vi "nominal workbook create commit.vi"(7 "out_workbook":i32, 8 "error in (no error)":errorcluster, 9 "staging":i32, 10 "template_":i32, 11 "client":i32) -> (0 "error out":errorcluster, 3 "function return":i32, 5 "out_workbook out":i32)   [LabVIEW 2020, in "client.lvlib"]
doc: "int32_t nominal_workbook_create_commit(int32_t client,\n int32_t template_,\n int32_t staging,\n int32_t *out_workbook);"
uses:
  client.lvlib
  bin/nominalClient_64.dll
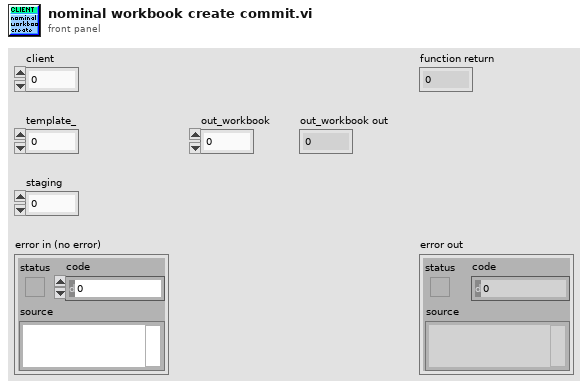
[diagram p1: front panel]
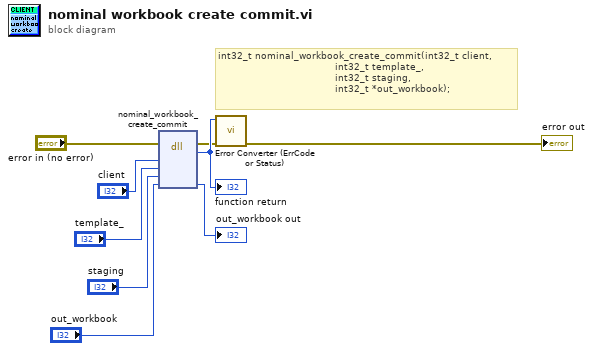
[diagram p0: block diagram]
diagram:
  # "int32_t nominal_workbook_create_commit(int32_t client,\n                                       int32_t template_,\n                                       int32_t staging,\n                                       int32_t *out_workbook);"
  n1 = dll-call lib="C:/code/labview-client-rs/lv_src/bin/nominalClient_*.*" fn="nominal_workbook_create_commit"(error in="error in (no error)", "client"="client", "template_"="template_", "staging"="staging", "out_workbook"="out_workbook") -> (error out=w2:errorcluster, w9:i32, "out_workbook"=→"out_workbook out":i32)  [unwired: 5 in, 1 out]
  "function return" <- w9
  n2 = call "Error Converter (ErrCode or Status).vi"("error in (no error)"=w2, "error code"=w9) -> ("error out"=→"error out":errorcluster)  [unwired: 9 in]
